vi "selectDecayRegion.vi"(4 "Cursor List":T1, 5 "only selected region?":bool, 6 "histogram 3":dbl[](array[numeric]), 7 "histogram 2":dbl[](array[numeric]), 8 "histogram 1":dbl[](array[numeric]), 9 "time in":dbl[](array[numeric])) -> (0 "histogram 3 out":dbl[](array[numeric]), 1 "histogram2 out":dbl[](array[numeric]), 2 "histogram 1 out":dbl[](array[numeric]), 3 "time out":dbl[](array[numeric]))   [LabVIEW 2009]
uses:
  <vilib>/Utility/miscctls.llb/LVCursorListTypeDef.ctl
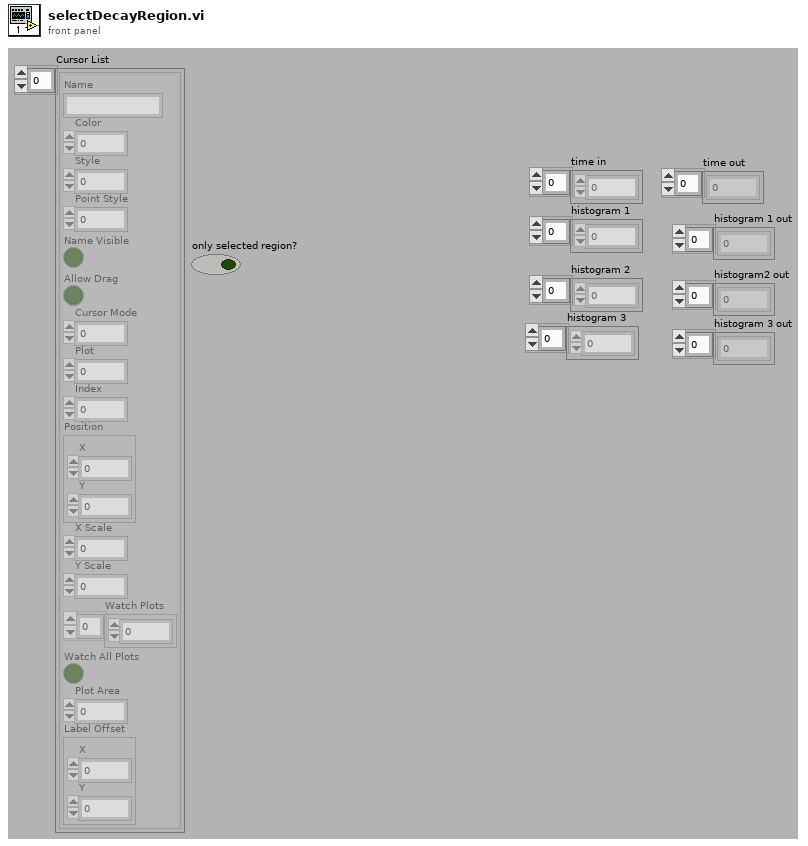
[diagram p1: front panel]
types:
  T1 = typedef "LVCursorListTypeDef.ctl" = cluster{"Name":string, "Color":u32, "Style":u8, "Point Style":u8, "Name Visible":bool, "Allow Drag":bool, "Cursor Mode":u32, "Plot":i32, "Index":i32, "Position":cluster{"X":dbl, "Y":dbl}, "X Scale":u32, "Y Scale":u32, "Watch Plots":i32[], "Watch All Plots":bool, "Plot Area":i32, "Label Offset":cluster{"X":dbl, "Y":dbl}}[]
  T2 = cluster{"Name":string, "Color":u32, "Style":u8, "Point Style":u8, "Name Visible":bool, "Allow Drag":bool, "Cursor Mode":u32, "Plot":i32, "Index":i32, "Position":cluster{"X":dbl, "Y":dbl}, "X Scale":u32, "Y Scale":u32, "Watch Plots":i32[], "Watch All Plots":bool, "Plot Area":i32, "Label Offset":cluster{"X":dbl, "Y":dbl}}
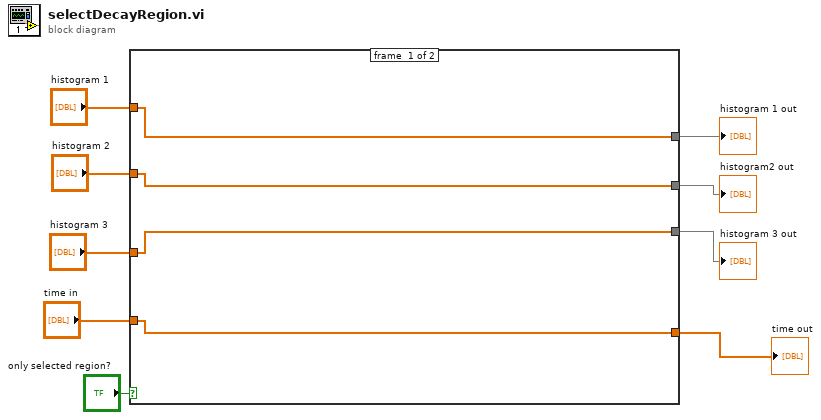
[diagram p0: block diagram]
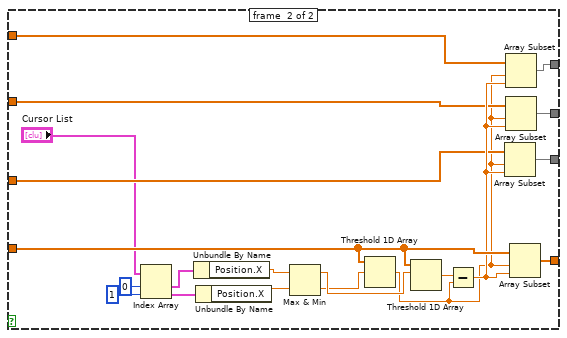
[diagram p2: hidden frame]
diagram:
  n1 = case shown="False" "only selected region?" {
    tunnel: "time in" -> [w10 w33]
    tunnel: "histogram 1" -> [w13 w23]
    tunnel: "histogram 2" -> [w12 w22]
    tunnel: "histogram 3" -> [w11 w21]
    tunnel: [w13 w20] -> w5
    tunnel: [w12 w19] -> w4
    tunnel: [w11 w18] -> w3
    tunnel: [w10 w15] -> w2
    frame #0 {
    }
    frame #1 {
      n2 = Index Array(array="Cursor List", index #1=0 ("Index"), index #2=1 ("Index")) -> (element #1=w27:T2, element #2=w28:T2)
      n3 = Unbundle By Name(w27) -> ("Position.X"=w29:dbl)
      n4 = Unbundle By Name(w28) -> ("Position.X"=w30:dbl)
      n5 = Max & Min(x=w29, y=w30) -> (max(x,y)=w32:dbl, min(x,y)=w31:dbl)
      n6 = Threshold 1D Array(2:w31, 3:w33) -> (0:w16:dbl)  [unwired: 1 in]
      n7 = Threshold 1D Array(2:w32, 3:w33) -> (0:w17:dbl)  [unwired: 1 in]
      n8 = Subtract(x=w17, y=w16) -> (x-y=w24:dbl)
      n9 = Array Subset(array=w21, index=w16, length=w24) -> (w18:dbl[])
      n10 = Array Subset(array=w23, index=w16, length=w24) -> (w20:dbl[])
      n11 = Array Subset(array=w22, index=w16, length=w24) -> (w19:dbl[])
      n12 = Array Subset(array=w33, index=w16, length=w24) -> (w15:dbl[])
    }
  }
  "time out" <- w2
  "histogram 1 out" <- w5
  "histogram2 out" <- w4
  "histogram 3 out" <- w3
